vi "Subvi_Training_Baseline_w_range_w_weight_1세부통합.vi"(4 "Nontarget_Flash_Order":i32[][](array[numeric]), 5 "Target_Flash_Order":i64[](array[numeric]), 6 "samples per channel":i32=25, 7 "Brain_data_source":dbl[][](array[numeric]) caption="EEG_Raw_Data" format="%0.3f", 8 "rate":dbl=500.0 caption="Rate" format="%0.2f", 9 "Experimentation_num":i32=2, 10 "Random_num":i32=9, 11 "Random_Repeat":i32=20) -> (0 "Target_ERP":dbl[][](array[numeric]), 1 "NonTarget":dbl[][](array[numeric]), 2 "Nontarget_ERP":dbl[][](array[numeric]), 3 "Target":dbl[][](array[numeric]))   [LabVIEW 2014]
uses:
  <vilib>/Analysis/3filter.llb/Filter Passband Type.ctl
  <vilib>/Analysis/baseanly.llb/Mean (DBL).vi
  <vilib>/Analysis/3filter.llb/Butterworth Filter (DBL).vi
  <vilib>/Analysis/NI_AALBase.lvlib
  <vilib>/Utility/file.llb/Read From Spreadsheet File (DBL).vi
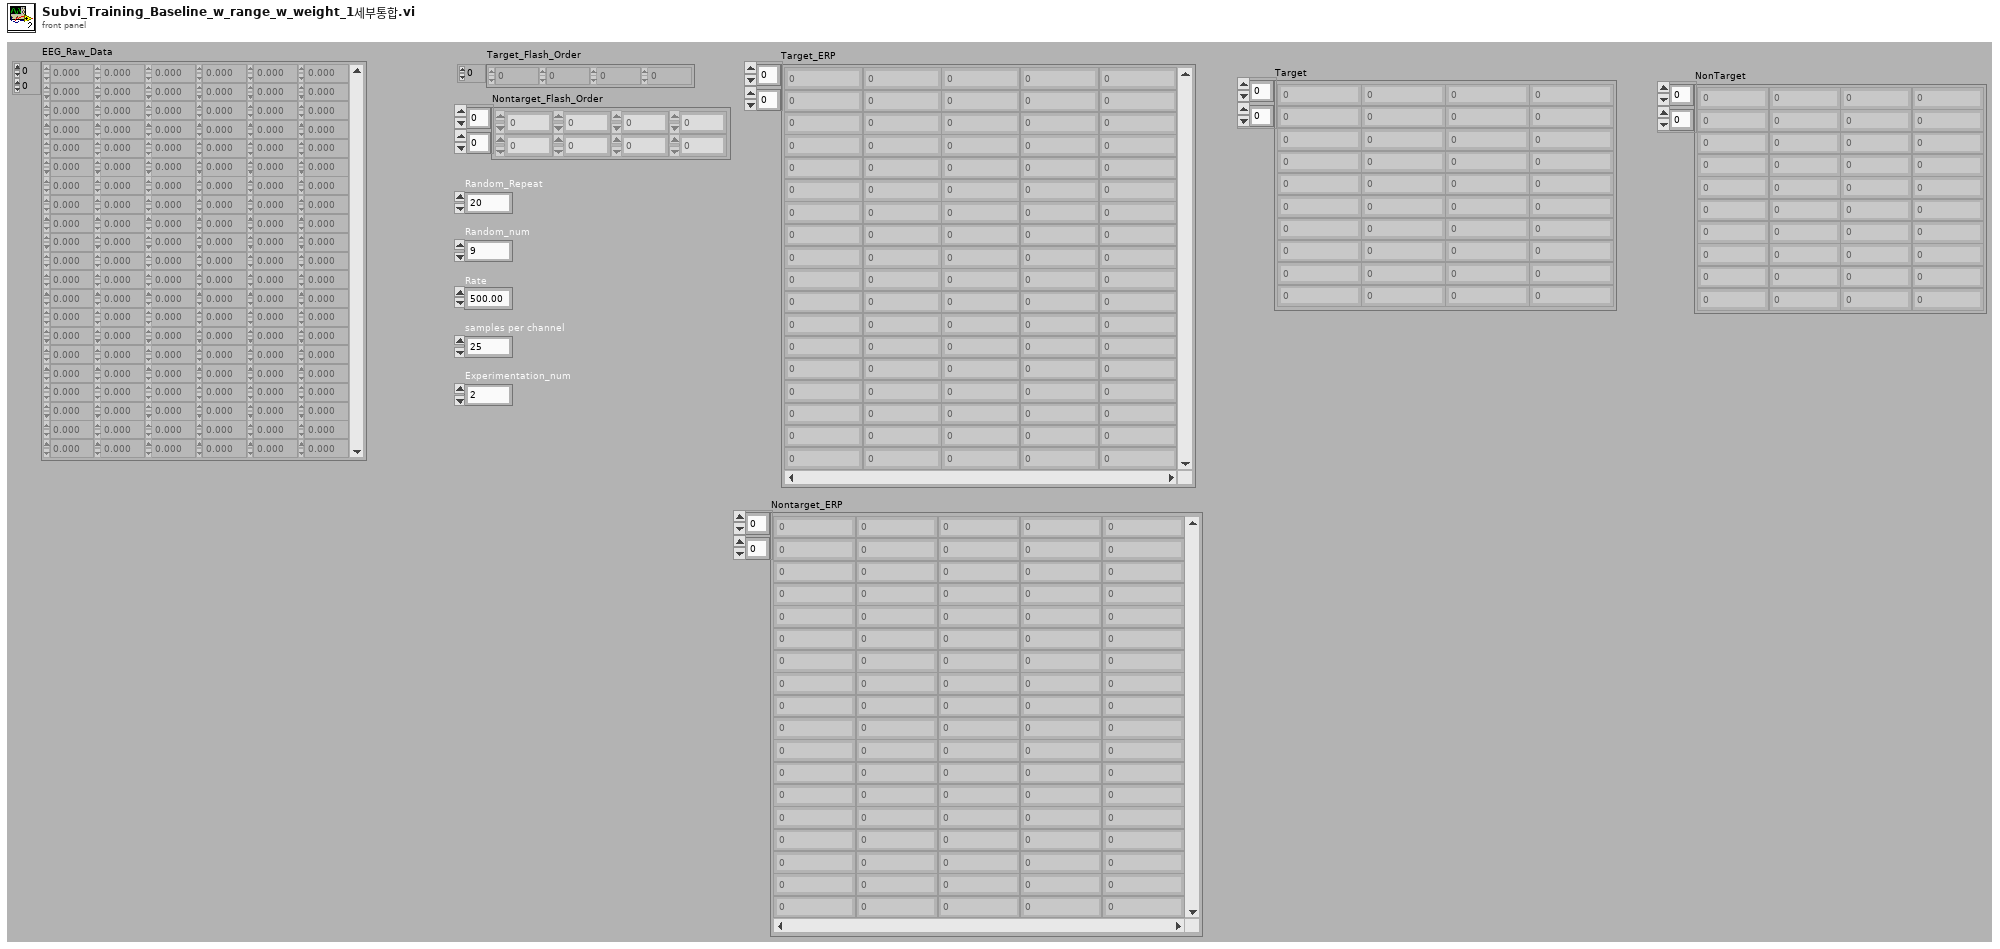
[diagram p1: front panel]
types:
  T1 = typedef "NI_AALBase.lvlib/Filter Passband Type.ctl" = enum32{"Lowpass", "Highpass", "Bandpass", "Bandstop"}
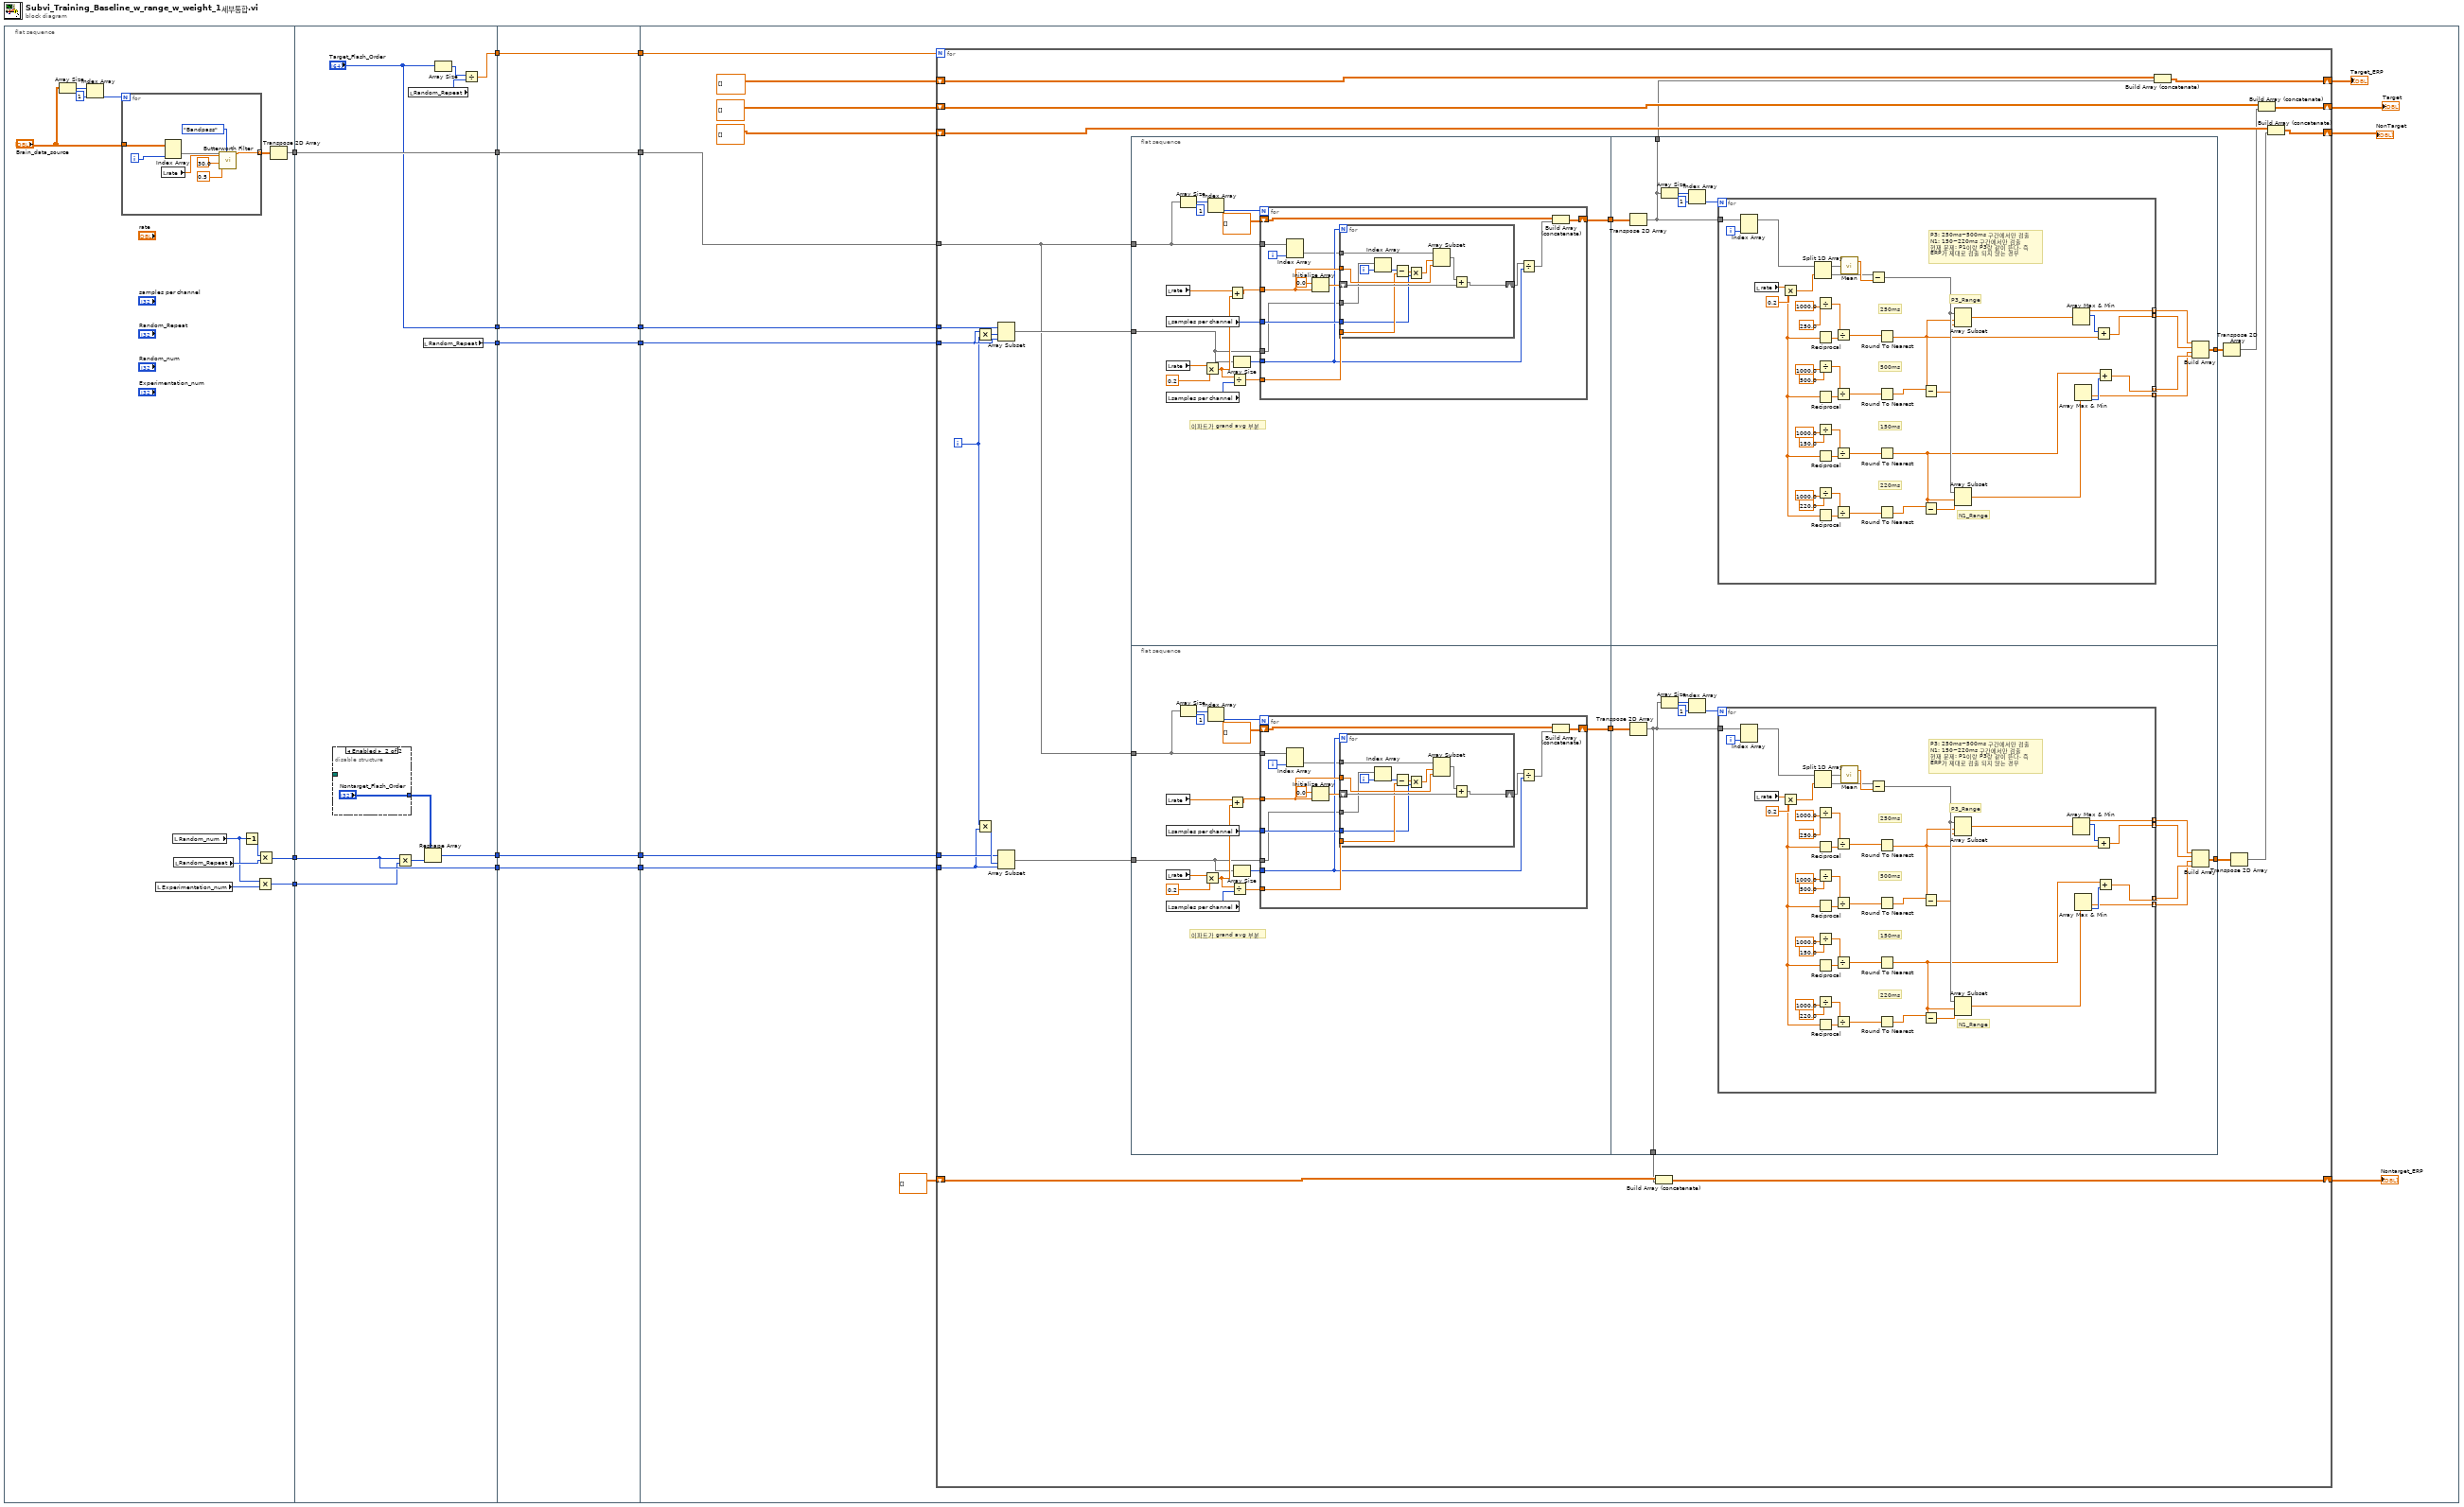
[diagram p0: block diagram]
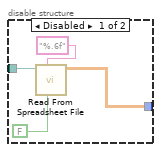
[diagram p2: hidden frame]
diagram:
  n1 = flat-sequence {
    tunnel: [w16] -> w15
    tunnel: [w25] -> w14
    tunnel: [w22] -> w13
    tunnel: w15 -> [w46]
    tunnel: [w46] -> w12
    tunnel: [w43] -> w10
    tunnel: ["Target_Flash_Order"] -> w8
    tunnel: [w42] -> w6
    tunnel: w14 -> [w39]
    tunnel: [w40] -> w4
    tunnel: [w39] -> w2
    tunnel: w13 -> [w38]
    tunnel: w12 -> [w52]
    tunnel: [w52] -> w11
    tunnel: w10 -> [w57]
    tunnel: [w57] -> w9
    tunnel: w8 -> [w56]
    tunnel: [w56] -> w7
    tunnel: w6 -> [w55]
    tunnel: [w55] -> w5
    tunnel: w4 -> [w54]
    tunnel: [w54] -> w3
    tunnel: w2 -> [w53]
    tunnel: [w53] -> w1
    tunnel: w11 -> [w71]
    tunnel: w9 -> [w62]
    tunnel: w7 -> [w70]
    tunnel: w5 -> [w69]
    tunnel: w3 -> [w68]
    tunnel: w1 -> [w67]
    frame #0 {
      n2 = Array Size(array="Brain_data_source") -> (size(s)=w20:i32[])
      n3 = Index Array(array=w20, index=1) -> (element=w18:i32)
      n4 = for {
        N: w18 -> [_]
        tunnel: "Brain_data_source" -> [w31]
        tunnel: [w30] -> w21 mode=indexing
        i -> [w28]
        n5 = local read "rate"() -> (w32:dbl)
        n6 = Index Array(array=w31, index (col)=w28) -> (element=w29:dbl[])  [unwired: 1 in]
        n7 = call-poly <vilib>:"Butterworth Filter.vi"("filter type"=Filter_Passband_Type."Bandpass", "low cutoff freq: fl"=0.5, "high cutoff freq: fh"=30.0, "sampling freq: fs"=w32, "X"=w29) -> ("Filtered X"=w30:dbl[])  [unwired: 3 in, 1 out]
      }
      n8 = local read "Experimentation_num"() -> (w24:i32)
      n9 = local read "Random_num"() -> (w23:i32)
      n10 = local read "Random_Repeat"() -> (w26:i32)
      n11 = Decrement(x=w23) -> (x-1=w27:i32)
      n12 = Multiply(x=w23, y=w24) -> (x*y=w22:i32)
      n13 = Multiply(x=w27, y=w26) -> (x*y=w25:i32)
      n14 = Transpose 2D Array(2D array=w21) -> (transposed array=w16:dbl[][])
    }
    frame #1 {
      n15 = disable-structure shown="Enabled" {
        disable-tunnel: _ -> [w50 _]
        disable-tunnel: [w48 "Nontarget_Flash_Order"] -> w37
        frame Disabled {
          n16 = call-poly <vilib>:"Read From Spreadsheet File.vi"("transpose (no:F)"=FALSE, "format (%.3f)"="%.6f", "file path (dialog if empty)"=w50) -> ("all rows"=w48:dbl[][])  [unwired: 4 in, 4 out]
        }
        frame Enabled {
        }
      }
      n17 = Multiply(x=w39, y=w38) -> (x*y=w41:i32)
      n18 = local read "Random_Repeat"() -> (w44:i32)
      n19 = local read "Random_Repeat"() -> (w42:i32)
      n20 = Reshape Array(w37, w41) -> (w40:i32[])
      n21 = Array Size(array="Target_Flash_Order") -> (size(s)=w45:i32)
      n22 = Divide(x=w45, y=w44) -> (x/y=w43:dbl)
    }
    frame #2 {
    }
    frame #3 {
      n23 = for {
        N: w62 -> [_]
        tunnel: w71 -> [w73]
        tunnel: w70 -> [w97]
        tunnel: w69 -> [w95]
        tunnel: w68 -> [w91]
        tunnel: w67 -> [w90]
        shift-right: [w88] -> w64
        shift-left: dbl[][] [] -> [w89]
        shift-right: [w87] -> w63
        shift-left: dbl[][] [] -> [w86]
        shift-right: [w83] -> w59
        shift-left: dbl[][] [] -> [w81]
        shift-right: [w84] -> w58
        shift-left: dbl[][] [] -> [w85]
        i -> [w92]
        n24 = Multiply(x=w95, y=w92) -> (x*y=w96:i32)
        n25 = Multiply(x=w92, y=w90) -> (x*y=w93:i32)
        n26 = Array Subset(array=w97, index=w96, length=w95) -> (w94:i64[])
        n27 = Array Subset(array=w91, index=w93, length=w90) -> (w74:i32[])
        n28 = flat-sequence {
          tunnel: w73 -> [w195]
          tunnel: w94 -> [w198]
          tunnel: [w193] -> w79
          tunnel: [w243] -> w80
          tunnel: [w238] -> w82
          tunnel: w79 -> [w242]
          frame #0 {
            (unwired) 1 ("index")
            # "이파트가 grand avg 부분"
            n29 = local read "rate"() -> (w205:dbl)
            n30 = local read "samples per channel"() -> (w200:i32)
            n31 = local read "rate"() -> (w203:dbl)
            n32 = local read "samples per channel"() -> (w201:i32)
            n33 = Array Size(array=w195) -> (size(s)=w197:i32[])
            n34 = Multiply(x=w203, y=0.2) -> (x*y=w207:dbl)
            n35 = Index Array(array=w197) -> (element=w196:i32)  [unwired: 1 in]
            n36 = Add(x=w205, y=w207) -> (x+y=w206:dbl)
            n37 = Divide(x=w207, y=w201) -> (x/y=w204:dbl)
            n38 = Array Size(array=w198) -> (size(s)=w199:i32)
            n39 = for {
              N: w196 -> [_]
              tunnel: w206 -> [w221]
              tunnel: w204 -> [w220]
              tunnel: w200 -> [w219]
              tunnel: w195 -> [w213]
              tunnel: w199 -> [w215]
              tunnel: w198 -> [w214]
              shift-right: [w209] -> w193
              shift-left: dbl[][] [] -> [w208]
              i -> [w212]
              n40 = Index Array(array=w213, index (col)=w212) -> (element=w211:dbl[])  [unwired: 1 in]
              n41 = Initialize Array(0.0 ("element"), w221) -> (w218:dbl[])
              n42 = for {
                N: w215 -> [_]
                shift-right: [w231] -> w216
                shift-left: w218 -> [w232]
                tunnel: w221 -> [w230]
                tunnel: w214 -> [w228]
                tunnel: w220 -> [w226]
                tunnel: w219 -> [w224]
                tunnel: w211 -> [w223]
                i -> [w229]
                n43 = Index Array(array=w228, index=w229) -> (element=w227:i64)
                n44 = Subtract(x=w227, y=w226) -> (x-y=w225:dbl)
                n45 = Multiply(x=w225, y=w224) -> (x*y=w233:dbl)
                n46 = Array Subset(array=w223, index=w233, length=w230) -> (w222:dbl[])
                n47 = Add(x=w222, y=w232) -> (x+y=w231:dbl[])
              }
              n48 = Divide(x=w216, y=w215) -> (x/y=w210:dbl[])
              n49 = Build Array (concatenate)(w208, w210) -> (w209:dbl[][])
            }
          }
          frame #1 {
            n50 = Transpose 2D Array(2D array=w242) -> (transposed array=w238:dbl[][])
            n51 = Array Size(array=w238) -> (size(s)=w240:i32[])
            n52 = Index Array(array=w240, index=1) -> (element=w239:i32)
            n53 = for {
              N: w239 -> [_]
              tunnel: w238 -> [w250]
              tunnel: [w247] -> w237 mode=indexing
              tunnel: [w246] -> w236 mode=indexing
              tunnel: [w245] -> w234 mode=indexing
              tunnel: [w244] -> w235 mode=indexing
              i -> [w248]
              # "N1_Range"
              # "P3_Range"
              # "220ms"
              # "150ms"
              # "500ms"
              # "250ms"
              # "P3: 250ms~500ms 구간에서만 검출\nN1: 150~220ms 구간에서만 검출\n현재 문제: P1이랑 P3랑 같이 뜬다. 즉\nERP가 제대로 검출 되지 않는 경우"
              n54 = Index Array(array=w250, index (col)=w248) -> (element=w249:dbl[])  [unwired: 1 in]
              n55 = local read "rate"() -> (w280:dbl)
              n56 = Multiply(x=w280, y=0.2) -> (x*y=w286:dbl)
              n57 = Split 1D Array(array=w249, index=w286) -> (first subarray=w285:dbl[], second subarray=w281:dbl[])
              n58 = Divide(x=250.0, y=1000.0) -> (x/y=w275:dbl)
              n59 = Reciprocal(x=w280) -> (1/x=w279:dbl)
              n60 = Divide(x=500.0, y=1000.0) -> (x/y=w274:dbl)
              n61 = Reciprocal(x=w280) -> (1/x=w278:dbl)
              n62 = Divide(x=150.0, y=1000.0) -> (x/y=w273:dbl)
              n63 = Reciprocal(x=w280) -> (1/x=w277:dbl)
              n64 = Divide(x=220.0, y=1000.0) -> (x/y=w272:dbl)
              n65 = Reciprocal(x=w280) -> (1/x=w276:dbl)
              n66 = Divide(x=w275, y=w279) -> (x/y=w263:dbl)
              n67 = Divide(x=w274, y=w278) -> (x/y=w262:dbl)
              n68 = Divide(x=w273, y=w277) -> (x/y=w261:dbl)
              n69 = Divide(x=w272, y=w276) -> (x/y=w260:dbl)
              n70 = call-poly <vilib>:"Mean.vi"("X"=w285) -> ("mean"=w284:dbl)  [unwired: 1 out]
              n71 = Subtract(x=w281, y=w284) -> (x-y=w257:dbl[])
              n72 = Round To Nearest(number=w263) -> (nearest integer value=w256:dbl)
              n73 = Round To Nearest(number=w262) -> (nearest integer value=w259:dbl)
              n74 = Round To Nearest(number=w261) -> (nearest integer value=w254:dbl)
              n75 = Round To Nearest(number=w260) -> (nearest integer value=w258:dbl)
              n76 = Subtract(x=w259, y=w256) -> (x-y=w255:dbl)
              n77 = Subtract(x=w258, y=w254) -> (x-y=w253:dbl)
              n78 = Array Subset(array=w257, index=w256, length=w255) -> (w252:dbl[])
              n79 = Array Subset(array=w257, index=w254, length=w253) -> (w251:dbl[])
              n80 = Array Max & Min(array=w252) -> (max value=w247:dbl, max index (indices)=w283:i32)  [unwired: 2 out]
              n81 = Array Max & Min(array=w251) -> (min value=w245:dbl, min index (indices)=w282:i32)  [unwired: 2 out]
              n82 = Add(x=w283, y=w256) -> (x+y=w246:dbl)
              n83 = Add(x=w254, y=w282) -> (x+y=w244:dbl)
            }
            n84 = Build Array(w237, w236, w234, w235) -> (w243:dbl[][])
          }
        }
        n85 = flat-sequence {
          tunnel: w73 -> [w100]
          tunnel: w74 -> [w103]
          tunnel: [w98] -> w76
          tunnel: [w148] -> w72
          tunnel: w76 -> [w147]
          tunnel: [w139] -> w75
          frame #0 {
            (unwired) 1 ("index")
            # "이파트가 grand avg 부분"
            n86 = local read "rate"() -> (w110:dbl)
            n87 = local read "samples per channel"() -> (w105:i32)
            n88 = local read "rate"() -> (w108:dbl)
            n89 = local read "samples per channel"() -> (w106:i32)
            n90 = Array Size(array=w100) -> (size(s)=w102:i32[])
            n91 = Multiply(x=w108, y=0.2) -> (x*y=w112:dbl)
            n92 = Index Array(array=w102) -> (element=w101:i32)  [unwired: 1 in]
            n93 = Add(x=w110, y=w112) -> (x+y=w111:dbl)
            n94 = Divide(x=w112, y=w106) -> (x/y=w109:dbl)
            n95 = Array Size(array=w103) -> (size(s)=w104:i32)
            n96 = for {
              N: w101 -> [_]
              tunnel: w111 -> [w126]
              tunnel: w109 -> [w125]
              tunnel: w105 -> [w124]
              tunnel: w100 -> [w118]
              tunnel: w104 -> [w120]
              tunnel: w103 -> [w119]
              shift-right: [w114] -> w98
              shift-left: dbl[][] [] -> [w113]
              i -> [w117]
              n97 = Index Array(array=w118, index (col)=w117) -> (element=w116:dbl[])  [unwired: 1 in]
              n98 = Initialize Array(0.0 ("element"), w126) -> (w123:dbl[])
              n99 = for {
                N: w120 -> [_]
                shift-right: [w136] -> w121
                shift-left: w123 -> [w137]
                tunnel: w126 -> [w135]
                tunnel: w119 -> [w133]
                tunnel: w125 -> [w131]
                tunnel: w124 -> [w129]
                tunnel: w116 -> [w128]
                i -> [w134]
                n100 = Index Array(array=w133, index=w134) -> (element=w132:i32)
                n101 = Subtract(x=w132, y=w131) -> (x-y=w130:dbl)
                n102 = Multiply(x=w130, y=w129) -> (x*y=w138:dbl)
                n103 = Array Subset(array=w128, index=w138, length=w135) -> (w127:dbl[])
                n104 = Add(x=w127, y=w137) -> (x+y=w136:dbl[])
              }
              n105 = Divide(x=w121, y=w120) -> (x/y=w115:dbl[])
              n106 = Build Array (concatenate)(w113, w115) -> (w114:dbl[][])
            }
          }
          frame #1 {
            n107 = Transpose 2D Array(2D array=w147) -> (transposed array=w139:dbl[][])
            n108 = Array Size(array=w139) -> (size(s)=w145:i32[])
            n109 = Index Array(array=w145, index=1) -> (element=w144:i32)
            n110 = for {
              N: w144 -> [_]
              tunnel: w139 -> [w155]
              tunnel: [w152] -> w143 mode=indexing
              tunnel: [w151] -> w142 mode=indexing
              tunnel: [w150] -> w140 mode=indexing
              tunnel: [w149] -> w141 mode=indexing
              i -> [w153]
              # "N1_Range"
              # "P3_Range"
              # "220ms"
              # "150ms"
              # "500ms"
              # "250ms"
              # "P3: 250ms~500ms 구간에서만 검출\nN1: 150~220ms 구간에서만 검출\n현재 문제: P1이랑 P3랑 같이 뜬다. 즉\nERP가 제대로 검출 되지 않는 경우"
              n111 = Index Array(array=w155, index (col)=w153) -> (element=w154:dbl[])  [unwired: 1 in]
              n112 = local read "rate"() -> (w185:dbl)
              n113 = Multiply(x=w185, y=0.2) -> (x*y=w191:dbl)
              n114 = Split 1D Array(array=w154, index=w191) -> (first subarray=w190:dbl[], second subarray=w186:dbl[])
              n115 = Divide(x=250.0, y=1000.0) -> (x/y=w180:dbl)
              n116 = Reciprocal(x=w185) -> (1/x=w184:dbl)
              n117 = Divide(x=500.0, y=1000.0) -> (x/y=w179:dbl)
              n118 = Reciprocal(x=w185) -> (1/x=w183:dbl)
              n119 = Divide(x=150.0, y=1000.0) -> (x/y=w178:dbl)
              n120 = Reciprocal(x=w185) -> (1/x=w182:dbl)
              n121 = Divide(x=220.0, y=1000.0) -> (x/y=w177:dbl)
              n122 = Reciprocal(x=w185) -> (1/x=w181:dbl)
              n123 = Divide(x=w180, y=w184) -> (x/y=w168:dbl)
              n124 = Divide(x=w179, y=w183) -> (x/y=w167:dbl)
              n125 = Divide(x=w178, y=w182) -> (x/y=w166:dbl)
              n126 = Divide(x=w177, y=w181) -> (x/y=w165:dbl)
              n127 = call-poly <vilib>:"Mean.vi"("X"=w190) -> ("mean"=w189:dbl)  [unwired: 1 out]
              n128 = Subtract(x=w186, y=w189) -> (x-y=w162:dbl[])
              n129 = Round To Nearest(number=w168) -> (nearest integer value=w161:dbl)
              n130 = Round To Nearest(number=w167) -> (nearest integer value=w164:dbl)
              n131 = Round To Nearest(number=w166) -> (nearest integer value=w159:dbl)
              n132 = Round To Nearest(number=w165) -> (nearest integer value=w163:dbl)
              n133 = Subtract(x=w164, y=w161) -> (x-y=w160:dbl)
              n134 = Subtract(x=w163, y=w159) -> (x-y=w158:dbl)
              n135 = Array Subset(array=w162, index=w161, length=w160) -> (w157:dbl[])
              n136 = Array Subset(array=w162, index=w159, length=w158) -> (w156:dbl[])
              n137 = Array Max & Min(array=w157) -> (max value=w152:dbl, max index (indices)=w188:i32)  [unwired: 2 out]
              n138 = Array Max & Min(array=w156) -> (min value=w150:dbl, min index (indices)=w187:i32)  [unwired: 2 out]
              n139 = Add(x=w188, y=w161) -> (x+y=w151:dbl)
              n140 = Add(x=w159, y=w187) -> (x+y=w149:dbl)
            }
            n141 = Build Array(w143, w142, w140, w141) -> (w148:dbl[][])
          }
        }
        n142 = Build Array (concatenate)(w85, w75) -> (w84:dbl[][])
        n143 = Build Array (concatenate)(w81, w82) -> (w83:dbl[][])
        n144 = Transpose 2D Array(2D array=w80) -> (transposed array=w78:dbl[][])
        n145 = Transpose 2D Array(2D array=w72) -> (transposed array=w77:dbl[][])
        n146 = Build Array (concatenate)(w89, w78) -> (w88:dbl[][])
        n147 = Build Array (concatenate)(w86, w77) -> (w87:dbl[][])
      }
      "Target" <- w64
      "NonTarget" <- w63
      "Target_ERP" <- w59
      "Nontarget_ERP" <- w58
    }
  }
